vi "Pre Launch Init.vi"(11 "Calibration Actor in":refnum<class "Calibration Actor.lvclass">) -> (0 "error out":errorcluster, 3 "Calibration Actor out":refnum<class "Calibration Actor.lvclass">)   [LabVIEW 2014, in "Calibration.lvlib" / "Calibration Actor.lvclass"]
doc: "(<B>Filename</B>: Actor Framework.lvlib:Actor.lvclass:Pre Launch Init.vi)\n\nDefines behavior that occurs after the Launch Nested Actor method is invoked but before the actor's Actor Core method begins running.\n\nBy default, this method does nothing. A descendant class may override it to define behavior."
uses:
  Calibration Actor.lvclass
  Calibration Actor.lvclass/Calibration Actor.ctl
  SuperActor/Read CVT Session.vi
  SuperActor/Ex Nested.lvclass
  <userlib>/_Session Fwk/Session - Root.lvclass
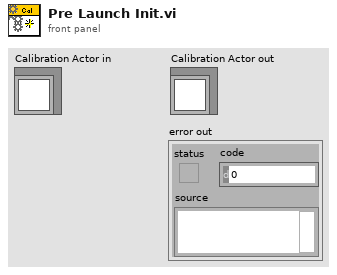
[diagram p1: front panel]
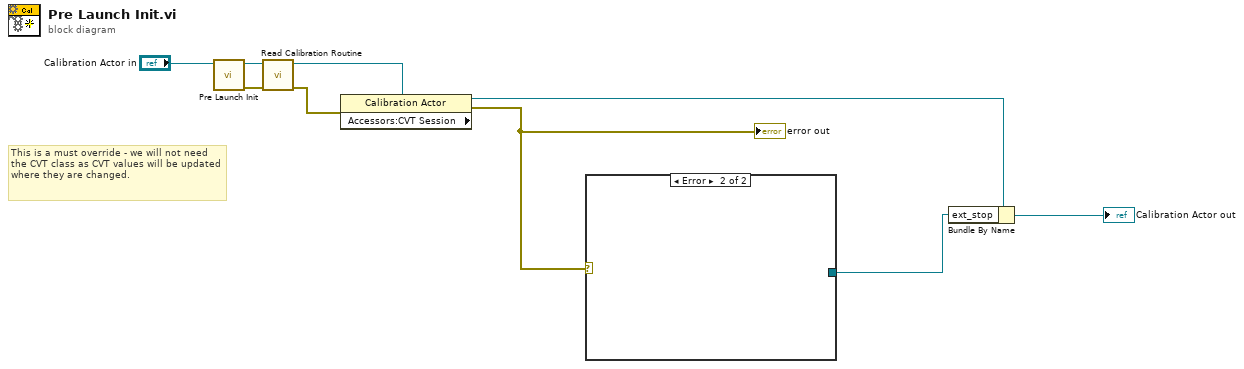
[diagram p0: block diagram]
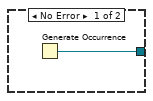
[diagram p2: hidden frame]
diagram:
  # "This is a must override - we will not need the CVT class as CVT values will be updated where they are changed."
  n1 = call-parent "Pre Launch Init.vi"("Ex Nested in"="Calibration Actor in") -> ("error out"=w7:errorcluster, "Ex Nested out"=w8:refnum<class "Calibration Actor.lvclass">)  [unwired: 9 in]
  n2 = call "Read Calibration Routine.vi"("error in"=w7, "Calibration Actor in"=w8) -> ("error out"=w5:errorcluster, "Calibration Actor out"=w6:refnum<class "Calibration Actor.lvclass">)  [unwired: 6 in, 2 out]
  n3 = property class="Calibration Actor" props=["Accessors:CVT Session"](reference=w6, error in=w5) -> (reference out=w3:refnum<class "Calibration Actor.lvclass">, error out=w4:errorcluster)  [unwired: 1 out]
  "error out" <- w4
  n4 = case shown="Error" w4 {
    tunnel: [w10 _] -> w1
    frame No Error {
      n5 = Generate Occurrence() -> (w10:refnum<k4>)
    }
    frame Error {
    }
  }
  n6 = Bundle By Name(cluster=w3, "ext_stop"=w1) -> (→"Calibration Actor out":refnum<class "Calibration Actor.lvclass">)
